vi "Format coverage report.vi"(0 "Not tested components":string[](array[string]), 1 "Not Tested position[x][y]":dbl[][](array[numeric]), 2 "Not Fitted position[x][y]":dbl[][](array[numeric]), 5 "TCF File path":path, 7 "Not fitted components":string[](array[string]), 9 "Program Name":string) -> (4 "Coverage text":string)   [LabVIEW 2013, in "Manipulate IPF.lvlib"]
uses:
  Manipulate IPF.lvlib
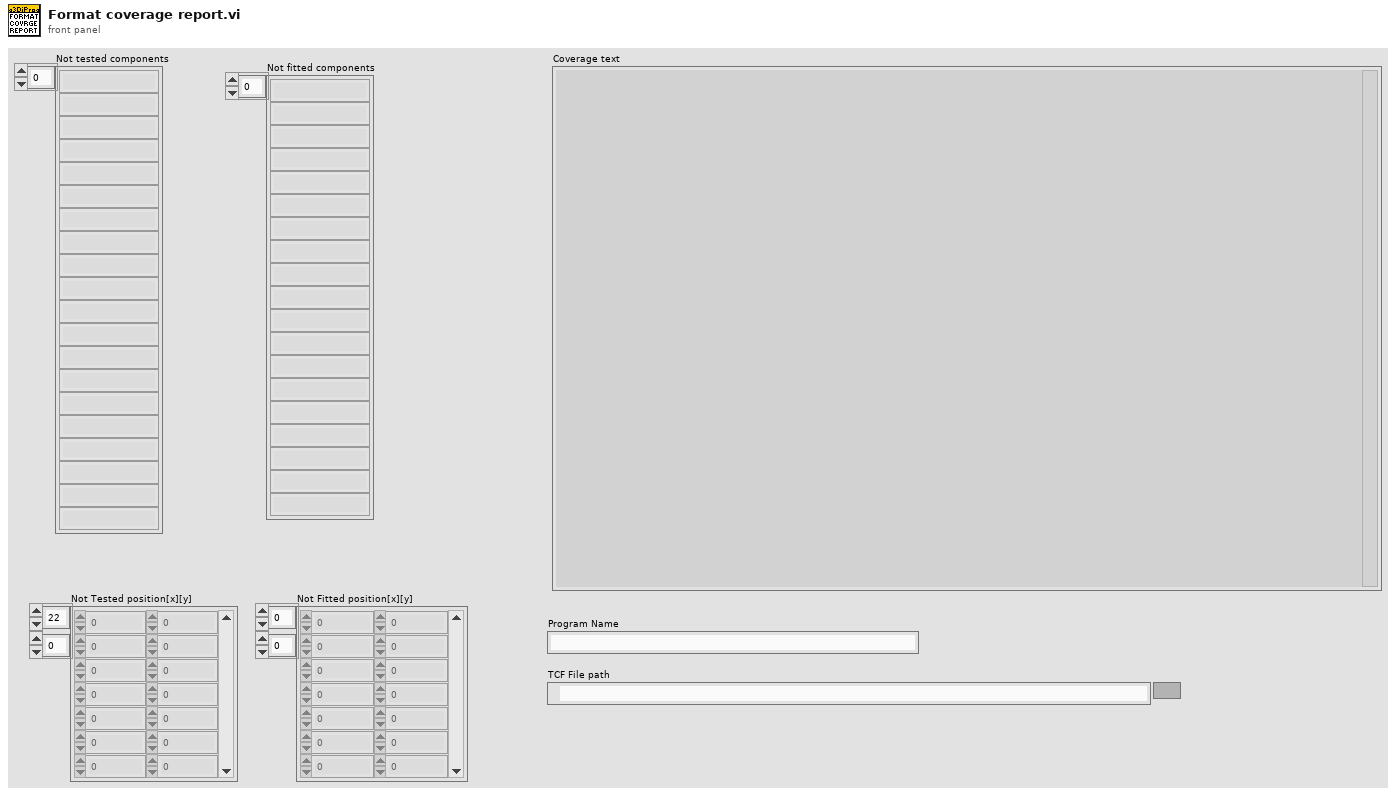
[diagram p1: front panel]
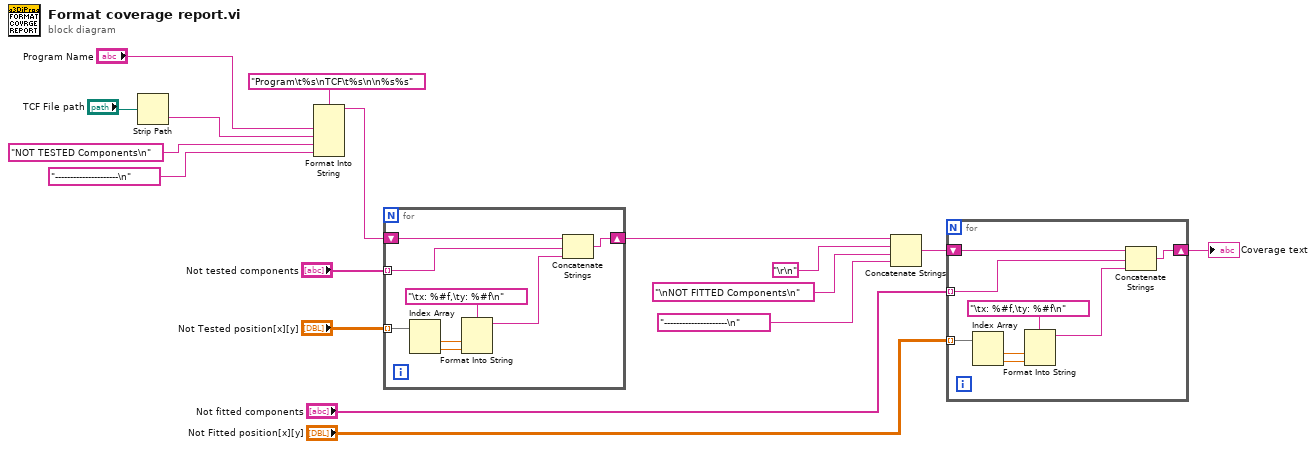
[diagram p0: block diagram]
diagram:
  n1 = Strip Path(path="TCF File path") -> (name=w6:string)  [unwired: 1 out]
  n2 = Format Into String(format string="Program\t%s\nTCF\t%s\n\n%s%s", "Program Name", w6, "NOT TESTED Components\n", "---------------------\n") -> (resulting string=w10:string)  [unwired: 2 in, 1 out]
  n3 = for {
    tunnel: "Not tested components" -> [w23] mode=indexing
    shift-right: [w24] -> w13
    shift-left: w10 -> [w25]
    tunnel: "Not Tested position[x][y]" -> [w18] mode=indexing
    n4 = Index Array(array=w18) -> (element #1=w22:dbl, element #2=w21:dbl)  [unwired: 2 in]
    n5 = Format Into String(format string="\tx: %#f,\ty: %#f\n", w22, w21) -> (resulting string=w20:string)  [unwired: 2 in, 1 out]
    n6 = Concatenate Strings(w25, w23, w20) -> (w24:string)
  }
  n7 = Concatenate Strings(w13, "\r\n", "\nNOT FITTED Components\n", "---------------------\n") -> (w4:string)
  n8 = for {
    tunnel: "Not fitted components" -> [w31] mode=indexing
    shift-right: [w32] -> w3
    shift-left: w4 -> [w33]
    tunnel: "Not Fitted position[x][y]" -> [w26] mode=indexing
    n9 = Index Array(array=w26) -> (element #1=w30:dbl, element #2=w29:dbl)  [unwired: 2 in]
    n10 = Format Into String(format string="\tx: %#f,\ty: %#f\n", w30, w29) -> (resulting string=w28:string)  [unwired: 2 in, 1 out]
    n11 = Concatenate Strings(w33, w31, w28) -> (w32:string)
  }
  "Coverage text" <- w3
